vi "HandleDoubleSolenoid.vi"() -> ()   [LabVIEW 2013]
uses:
  DoubleSolenoidAction.ctl
panel:
  in  "InitState":T1=enum."Middle"
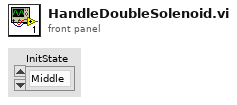
[diagram p1: front panel]
types:
  T1 = typedef "DoubleSolenoidAction.ctl" = enum16{"Init", "Out", "In", "Middle"}
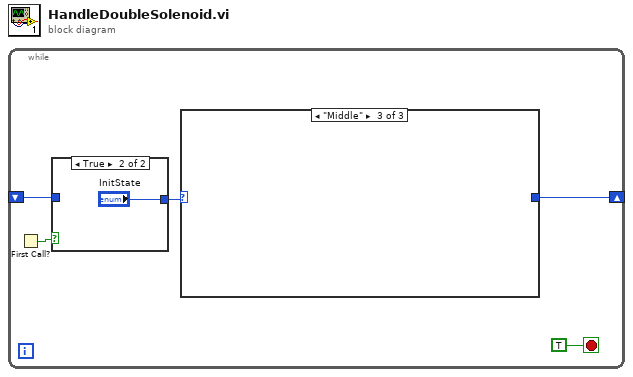
[diagram p0: block diagram]
diagram:
  n1 = while {
    shift-right: [w2] -> _
    shift-left: _ -> [w1]
    stop <- TRUE stop-if-true
    n2 = First Call?() -> (First Call?: T/F=w4:bool)
    n3 = case shown="True" w4 {
      tunnel: [w6 "InitState"] -> w3
      tunnel: w1 -> [w6 _]
      frame False {
      }
      frame True {
      }
    }
    n4 = case shown="\"Middle\"" w3 {
      selector: w3 -> [w8 _ _]
      tunnel: [w8 _ _] -> w2
      frame "Out" {
      }
      frame "In" {
      }
      frame "Middle" {
      }
    }
  }
